vi "Set Scanner.vi"(8 "error in (no error)":errorcluster, 10 "Scanner Settings":T1={"Scan1"=1, "Scan2"=1, "Scan3"=1, "Scan4"=1, "Scan5"=1, "Scan6"=1, "Scan7"=1, "Scan8"=1, "Scan9"=1, "Scan10"=1, "Scan11"=1, "Scan12"=1, "Scan13"=1, "Scan14"=1, "Scan15"=1, "Scan16"=1} {"Scan16" scale=0.0..2.0; "Scan15" scale=0.0..2.0; "Scan14" scale=0.0..2.0; "Scan13" scale=0.0..2.0; "Scan12" scale=0.0..2.0; "Scan11" scale=0.0..2.0; "Scan10" scale=0.0..2.0; "Scan9" scale=0.0..2.0; "Scan8" scale=0.0..2.0; "Scan7" scale=0.0..2.0; "Scan6" scale=0.0..2.0; "Scan5" scale=0.0..2.0; "Scan4" scale=0.0..2.0; "Scan3" min=0 max=2 scale=0.0..2.0; "Scan2" min=0 max=2 scale=0.0..2.0; "Scan1" min=0 max=2 scale=0.0..2.0}, 11 "VISA resource name":refnum<visa-resource-name>) -> (0 "error out":errorcluster, 3 "VISA resource name out":refnum<visa-resource-name>)   [LabVIEW 2020, in "Associated Research 78XX Series.lvlib"]
uses:
  <instrlib>/Associated Research 78XX Series/Associated Research 78XX Series.lvlib
  <instrlib>/Associated Research 78XX Series/Public/Configure/Steps/Low Level/Scanner Settings.ctl
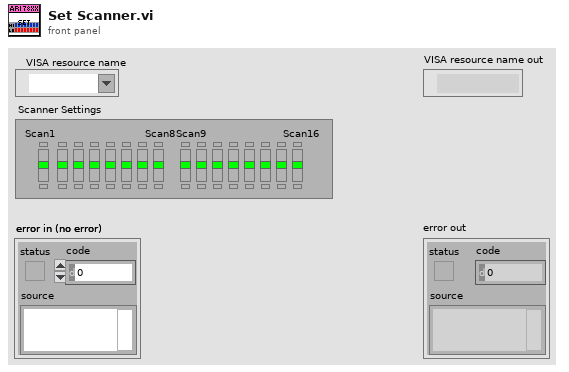
[diagram p1: front panel]
types:
  T1 = typedef "Associated Research 78XX Series.lvlib/Scanner Settings.ctl" = cluster{"Scan1":i32, "Scan2":i32, "Scan3":i32, "Scan4":i32, "Scan5":i32, "Scan6":i32, "Scan7":i32, "Scan8":i32, "Scan9":i32, "Scan10":i32, "Scan11":i32, "Scan12":i32, "Scan13":i32, "Scan14":i32, "Scan15":i32, "Scan16":i32}
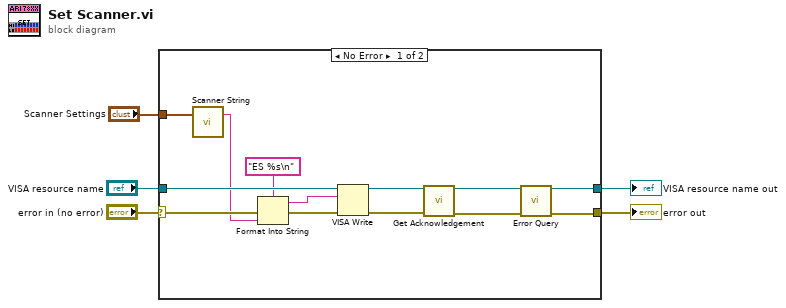
[diagram p0: block diagram]
diagram:
  n1 = case shown="No Error" "error in (no error)" {
    selector: "error in (no error)" -> [w16 w20]
    tunnel: [w15 w20] -> w4
    tunnel: [w17 w19] -> w2
    tunnel: "VISA resource name" -> [w18 w19]
    tunnel: "Scanner Settings" -> [w7 _]
    frame No Error {
      n2 = call <instrlib>:"Scanner String.vi"("Scanner Settings in"=w7) -> ("Scanner String (out)"=w6:string)  [unwired: 1 in, 1 out]
      n3 = Format Into String(format string="ES %s\n" ("\"False\" Command"), error in=w16, w6) -> (resulting string=w10:string, error out=w13:errorcluster)  [unwired: 1 in]
      n4 = VISA Write(VISA resource name=w18, write buffer=w10, error in (no error)=w13) -> (VISA resource name out=w9:refnum<visa-resource-name>, error out=w8:errorcluster)  [unwired: 1 out]
      n5 = call <instrlib>:"Get Acknowledgement.vi"("VISA resource name"=w9, "error in (no error)"=w8) -> ("VISA resource name out"=w12:refnum<visa-resource-name>, "error out"=w11:errorcluster)  [unwired: 12 in]
      n6 = call <instrlib>:"Error Query.vi"("VISA resource name"=w12, "error in (no error)"=w11) -> ("VISA resource name out"=w17:refnum<visa-resource-name>, "error out"=w15:errorcluster)  [unwired: 10 in, 2 out]
    }
    frame Error {
    }
  }
  "error out" <- w4
  "VISA resource name out" <- w2
